vi "Heat Up Check Range.vi"(11 "Array":dbl[](array[numeric])) -> (2 "Ouput Data":dbl[](array[numeric]), 3 "Add This Row":bool)   [LabVIEW 2019]
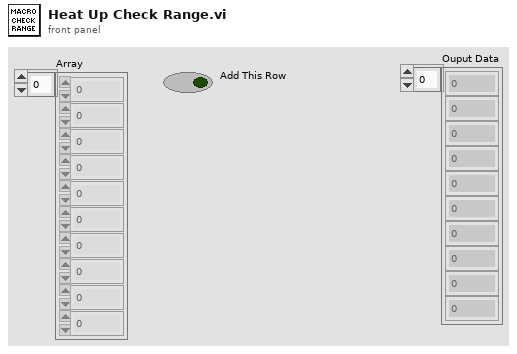
[diagram p1: front panel]
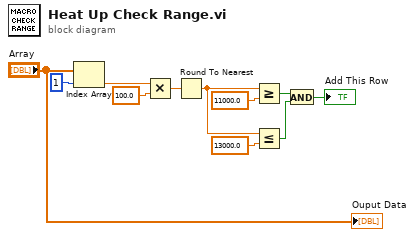
[diagram p0: block diagram]
diagram:
  n1 = Index Array(array="Array", index=1) -> (element=w9:dbl)
  n2 = Multiply(x=w9, y=100.0) -> (x*y=w11:dbl)
  n3 = Round To Nearest(number=w11) -> (nearest integer value=w7:dbl)
  n4 = Greater Or Equal?(x=w7, y=11000.0) -> (x >= y?=w3:bool)
  n5 = Less Or Equal?(x=w7, y=13000.0) -> (x <= y?=w5:bool)
  n6 = And(x=w3, y=w5) -> (x .and. y?=→"Add This Row":bool)
  "Ouput Data" <- "Array"
